vi "Begin.vi"() -> ()   [LabVIEW 2019]
doc: "Called before other user functions, this VI is expected to open initial I/O refnums, load in file data, and do all program initialization. Notice that the <B>error out</B> terminal is simply used for data flow. Wiring it to other structures or subVIs ensures that this VI runs first."
uses:
  <vilib>/Rock Robotics/WPI/Solenoid/WPI_SolenoidOpenSingle.vi
  <vilib>/Rock Robotics/WPI/RobotDrive/WPI_RobotDriveOpen4MotorWithSPARK.vi
  <vilib>/Rock Robotics/WPI/MotorControl/WPI_MotorControlOpen SPARK.vi
  <vilib>/Rock Robotics/WPI/MotorControl/WPI_MotorControlOpen TalonSRX.vi
  <vilib>/Rock Robotics/SystemInterfaces/DIO/FPGA_DIOPWMChannel.ctl
  <vilib>/Rock Robotics/WPI/Solenoid/WPI_SolenoidChannel.ctl
  <vilib>/Rock Robotics/WPI/Joystick/WPI_JoystickDeviceEnum.ctl
panel:
  in  "Shooting Motor 2 PWM Channel":T1
  in  "Shooting Motor 1 PWM Channel":T1
  in  "Peripherals Controller":T2
  in  "Drive Controller":T2
  in  "Transport Motor PWM Channel":T1
  in  "Intake Motor PWM Channel":T1
  in  "Pneumatics Control Module (0) 3":u8
  in  "Solenoid Channel 2":T3
  in  "Pneumatics Control Module (0) 2":u8
  in  "Solenoid Channel":T3
  in  "Pneumatics Control Module (0)":u8
  in  "Rear Camera Address":string="192.168.0.90"
  in  "Front Camera Address":string="192.168.0.90"
  in  "Front Right Motor Inverted":bool
  in  "Front Left Motor Inverted":bool
  in  "Rear Right Motor Inverted":bool
  in  "Rear Left Motor Inverted":bool
  in  "Front Right Motor":T1=enum."Invalid"
  in  "Front Left Motor":T1=enum."Invalid"
  in  "Rear Right Motor":T1=enum."Invalid"
  in  "Rear Left Motor":T1=enum."Invalid"
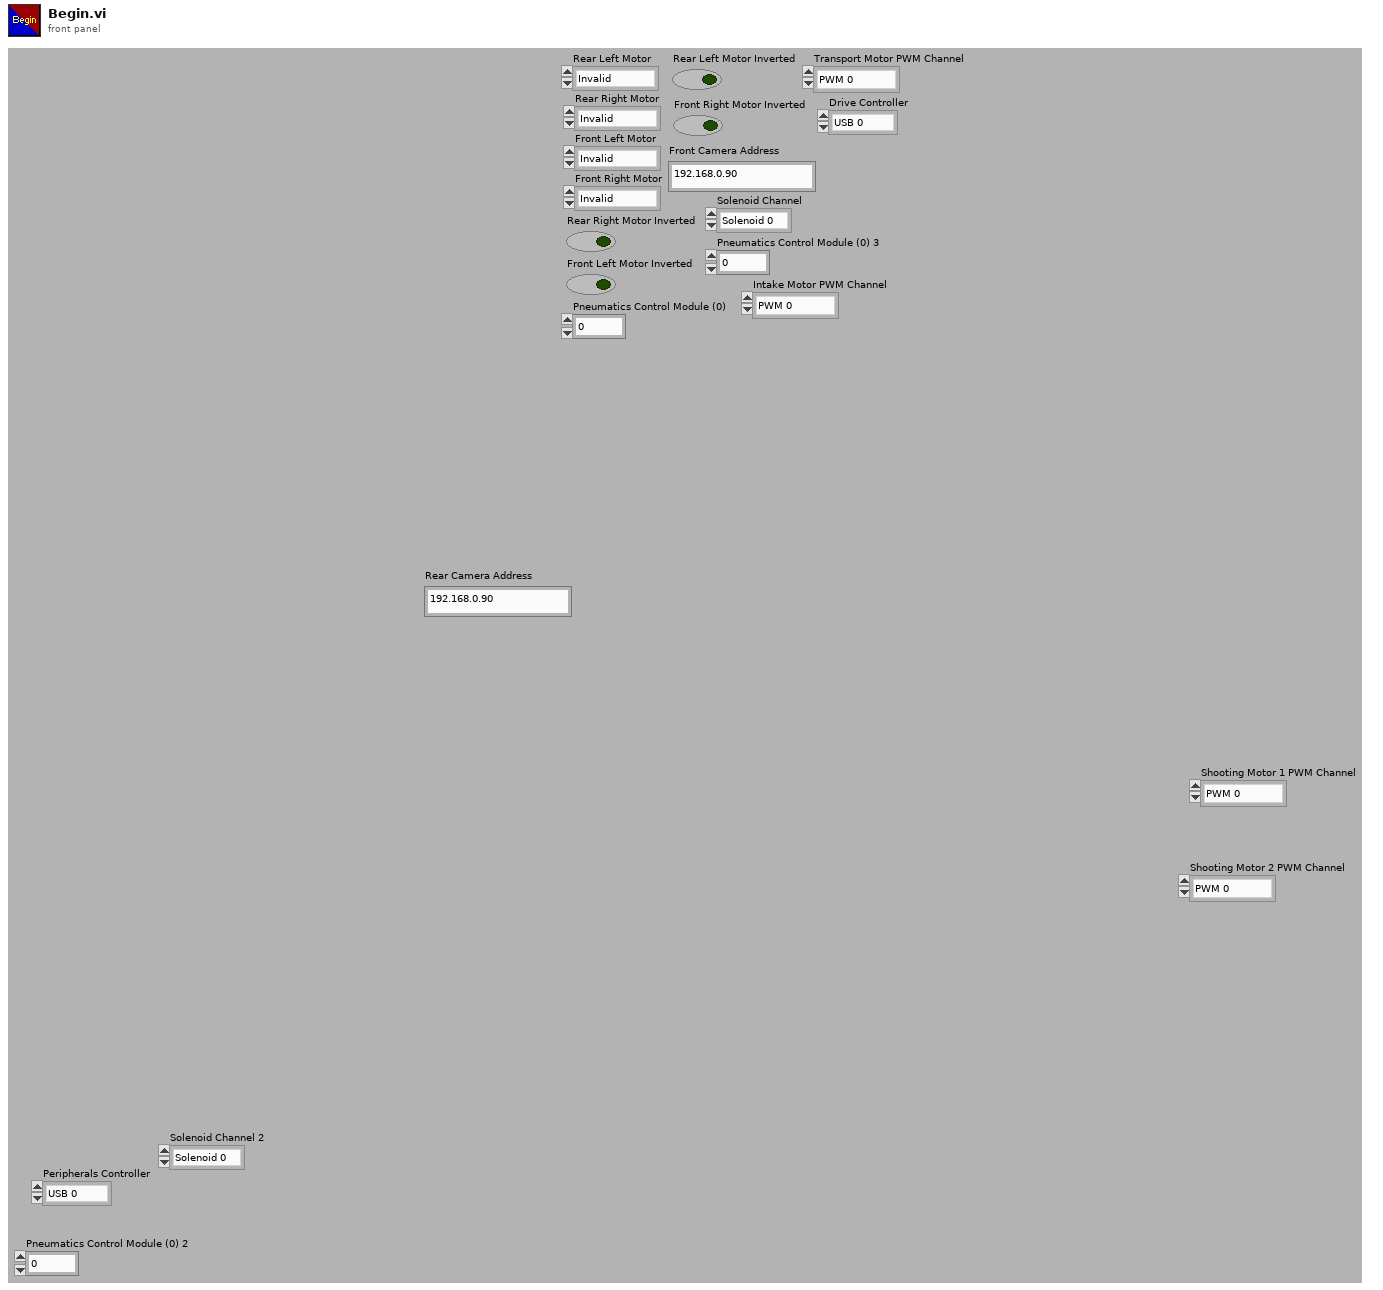
[diagram p1: front panel]
types:
  T1 = typedef "FPGA_DIOPWMChannel.ctl" = enum8{"PWM 0", "PWM 1", "PWM 2", "PWM 3", "PWM 4", "PWM 5", "PWM 6", "PWM 7", "PWM 8", "PWM 9", "PWM MXP 0", "PWM MXP 1", "PWM MXP 2", "PWM MXP 3", "PWM MXP 4", "PWM MXP 5", "PWM MXP 6", "PWM MXP 7", "PWM MXP 8", "PWM MXP 9", "Invalid"}
  T2 = typedef "WPI_JoystickDeviceEnum.ctl" = enum16{"USB 0", "USB 1", "USB 2", "USB 3", "USB 4", "USB 5"}
  T3 = typedef "WPI_SolenoidChannel.ctl" = enum8{"Solenoid 0", "Solenoid 1", "Solenoid 2", "Solenoid 3", "Solenoid 4", "Solenoid 5", "Solenoid 6", "Solenoid 7", "Invalid"}
  T4 = typedef "WPI_JoystickDevRef.ctl" = cluster{"Device":T2}
  T5 = typedef "WPI_RobotDriveDevRef.ctl" = cluster{"DevStatus":errorcluster, "Motors[]":T6[], "Square Inputs":bool, "Max Output":dbl}
  T6 = typedef "WPI_MotorControlDeviceRef.ctl" = cluster{"DeviceStatus":errorcluster, "Type":T7, "PWM":cluster{"PWM Channel":T1, "DeadBand":T8}, "CAN":cluster{"Device Number":u8, "SetOutput VI Ref":variant, "GetOutput VI Ref":variant, "Enable VI Ref":variant, "Disable VI Ref":variant, "Data":variant}, "Invert":bool, "DIO PWM":cluster{"PWM \"Enable\" Channel":T1, "DIOChannel":T9, "PWM Rate":dbl}}
  T7 = typedef "WPI_MotorControlType.ctl" = enum16{"PWM", "CAN", "DIO PWM"}
  T8 = typedef "WPI_PWMDeadband.ctl" = cluster{"Name":string, "maxPositivePwm":i32, "minPositivePwm":i32, "centerPwm":i32, "maxNegativePwm":i32, "minNegativePwm":i32, "angularRange":u16}
  T9 = typedef "FPGA_DIOChannel.ctl" = enum8{"DIO 0", "DIO 1", "DIO 2", "DIO 3", "DIO 4", "DIO 5", "DIO 6", "DIO 7", "DIO 8", "DIO 9", "DIO MXP 0", "DIO MXP 1", "DIO MXP 2", "DIO MXP 3", "DIO MXP 4", "DIO MXP 5", "DIO MXP 6", "DIO MXP 7", "DIO MXP 8", "DIO MXP 9", "DIO MXP 10", "DIO MXP 11", "DIO MXP 12", "DIO MXP 13", "DIO MXP 14", "DIO MXP 15", "SPI Port CS1", "SPI Port CS2", "SPI Port CS3", "SPI Port MISO", "SPI Port MOSI", "Invalid"}
  T10 = typedef "WPI_CameraDevRef.ctl" = cluster{"Camera Address":string, "CameraStatus":errorcluster}
  T11 = typedef "WPI_SolenoidDevRef.ctl" = cluster{"DevStatus":errorcluster, "Pneumatics Control Module":u8, "Forward Solenoid Channel":T3, "Reverse Solenoid Channel":T3}
  T12 = typedef "WPI_CompressorDevRef.ctl" = cluster{"DevStatus":errorcluster, "Pneumatics Control Module":u8}
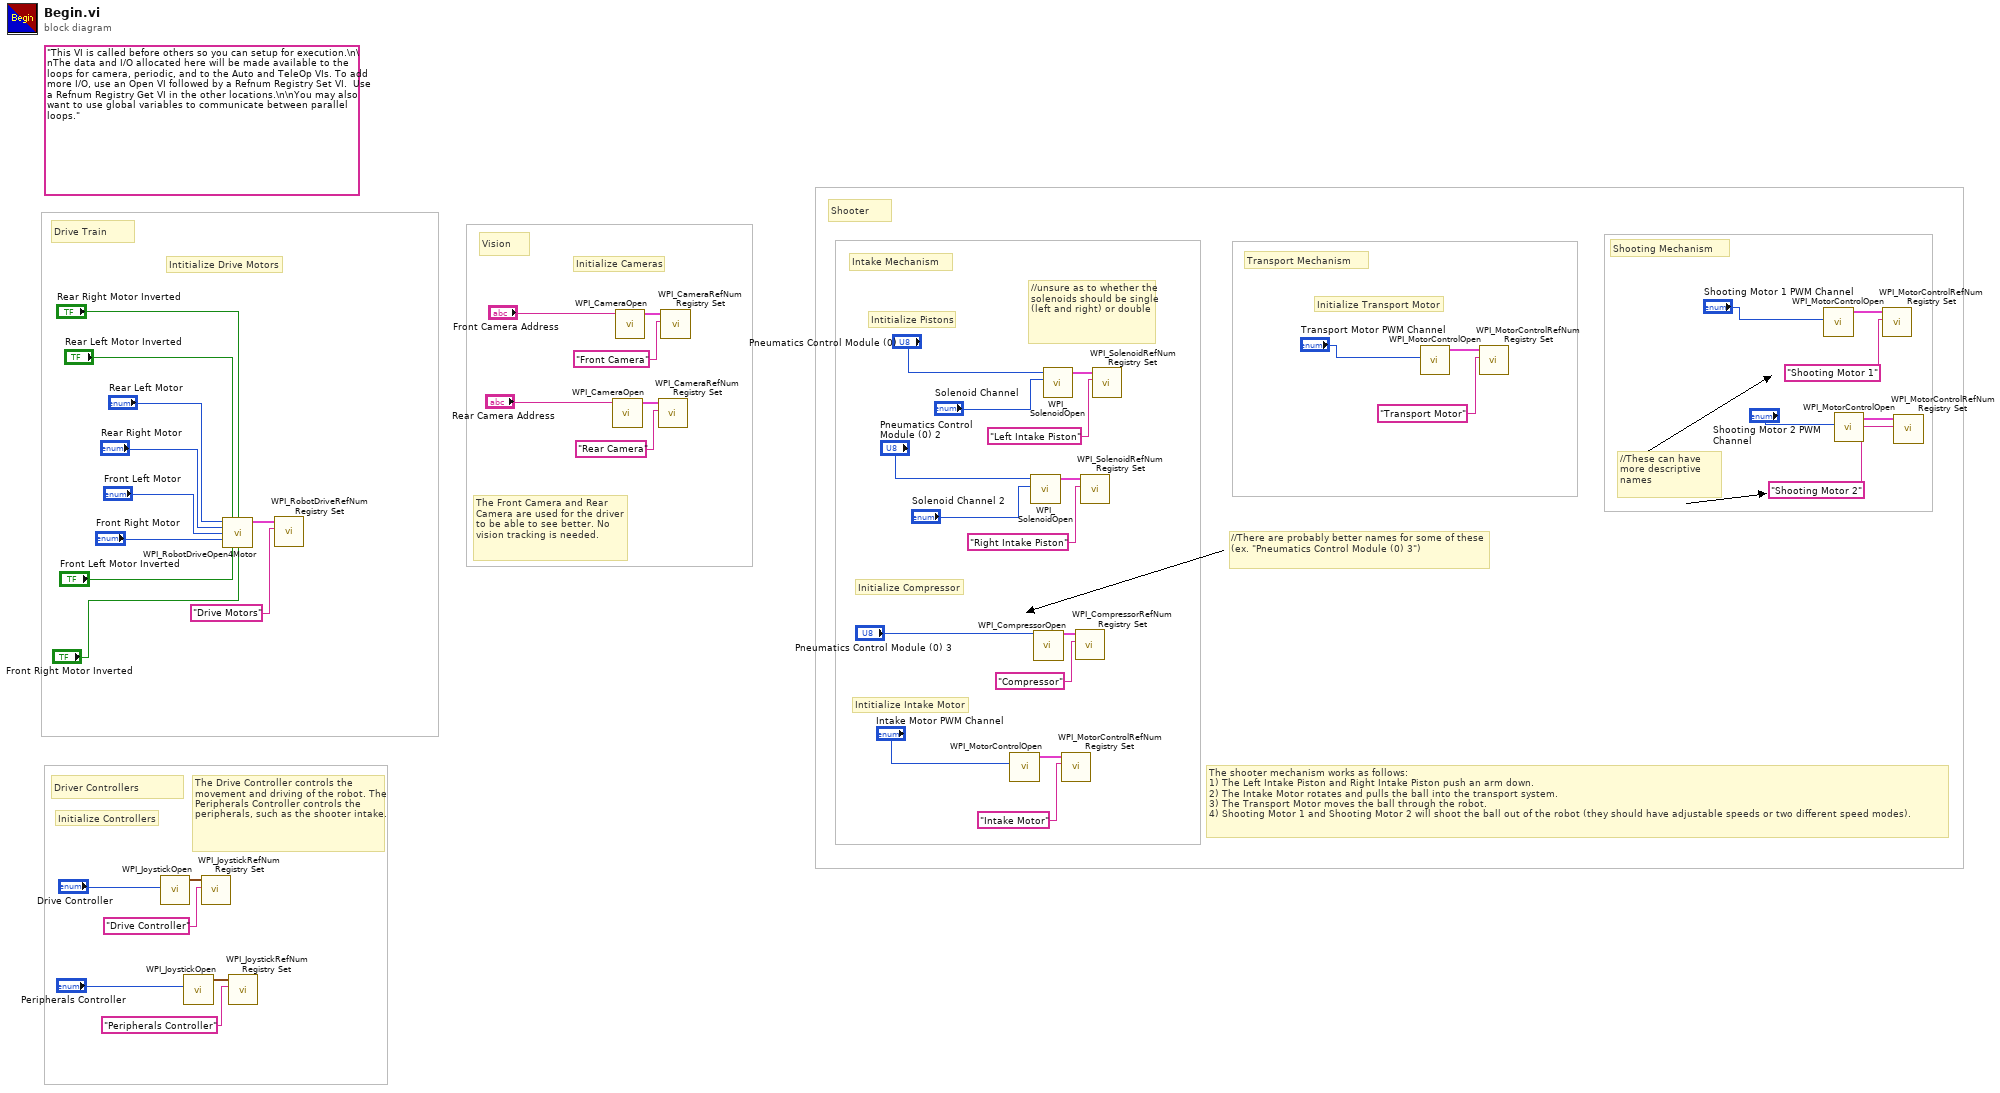
[diagram p0: block diagram]
diagram:
  (unwired) "This VI is called before others so you can setup for execution.\n\nThe data and I/O allocated here will be made available to the loops for camera, periodic, and to the Auto and TeleOp VIs. To add more I/O, use an Open VI followed by a Refnum Registry Set VI.  Use a Refnum Registry Get VI in the other locations.\n\nYou may also want to use global variables to communicate between parallel loops."
  # "Shooting Mechanism"
  # "//These can have more descriptive names"
  # "//unsure as to whether the solenoids should be single (left and right) or double"
  # "The shooter mechanism works as follows:\n1) The Left Intake Piston and Right Intake Piston push an arm down.\n2) The Intake Motor rotates and pulls the ball into the transport system.\n3) The Transport Motor moves the ball through the robot.\n4) Shooting Motor 1 and Shooting Motor 2 will shoot the ball out of the robot (they should have adjustable speeds or two different speed modes)."
  # "The Front Camera and Rear Camera are used for the driver to be able to see better. No vision tracking is needed."
  # "The Drive Controller controls the movement and driving of the robot. The Peripherals Controller controls the peripherals, such as the shooter intake."
  # "Initialize Controllers"
  # "Driver Controllers"
  # "//There are probably better names for some of these (ex. \"Pneumatics Control Module (0) 3\")"
  # "Transport Mechanism"
  # "Intake Mechanism"
  # "Shooter"
  # "Vision"
  # "Drive Train"
  # "Initialize Transport Motor"
  # "Intitialize Intake Motor"
  # "Initialize Compressor"
  # "Intitialize Pistons"
  # "Initialize Cameras"
  # "Intitialize Drive Motors"
  n1 = call <vilib>:"WPI_JoystickOpen.vi"("JoystickDevice"="Drive Controller") -> ("JoystickDevRef"=w12:T4)  [unwired: 10 in]
  n2 = call <vilib>:"WPI_JoystickOpen.vi"("JoystickDevice"="Peripherals Controller") -> ("JoystickDevRef"=w9:T4)  [unwired: 10 in]
  n3 = call <vilib>:"WPI_JoystickRefNum Registry Set.vi"("refnum name"="Drive Controller", "JoystickDevRef"=w12) -> ()  [unwired: 8 in, 2 out]
  n4 = call-poly <vilib>:"WPI_RobotDriveOpen4Motor.vi"("Rear Left Motor"="Rear Left Motor", "Rear Left Motor Inverted"="Rear Left Motor Inverted", "Rear Right Motor Inverted"="Rear Right Motor Inverted", "Rear Right Motor"="Rear Right Motor", "Front Left Motor"="Front Left Motor", "Front Right Motor"="Front Right Motor", "Front Left Motor Inverted"="Front Left Motor Inverted", "Front Right Motor Inverted"="Front Right Motor Inverted") -> ("RobotDriveDevRef"=w37:T5)  [unwired: 6 in, 1 out]
  n5 = call <vilib>:"WPI_JoystickRefNum Registry Set.vi"("refnum name"="Peripherals Controller", "JoystickDevRef"=w9) -> ()  [unwired: 8 in, 2 out]
  n6 = call <vilib>:"WPI_RobotDriveRefNum Registry Set.vi"("refnum name"="Drive Motors", "RobotDriveDevRef"=w37) -> ()  [unwired: 8 in, 2 out]
  n7 = call <vilib>:"WPI_CameraOpen.vi"("Camera Address"="Rear Camera Address") -> ("CameraDevRef"=w31:T10)  [unwired: 9 in, 1 out]
  n8 = call <vilib>:"WPI_CameraOpen.vi"("Camera Address"="Front Camera Address") -> ("CameraDevRef"=w34:T10)  [unwired: 9 in, 1 out]
  n9 = call <vilib>:"WPI_CameraRefNum Registry Set.vi"("refnum name"="Rear Camera", "CameraDevRef"=w31) -> ()  [unwired: 8 in, 2 out]
  n10 = call <vilib>:"WPI_CameraRefNum Registry Set.vi"("refnum name"="Front Camera", "CameraDevRef"=w34) -> ()  [unwired: 8 in, 2 out]
  n11 = call-poly <vilib>:"WPI_MotorControlOpen.vi"("PWM Channel"="Intake Motor PWM Channel") -> ("MotorControlDeviceRef"=w18:T6)  [unwired: 9 in, 1 out]
  n12 = call-poly <vilib>:"WPI_SolenoidOpen.vi"("Solenoid Channel"="Solenoid Channel 2", "Pneumatics Control Module (0)"="Pneumatics Control Module (0) 2") -> ("SolenoidDevRef"=w25:T11)  [unwired: 8 in, 1 out]
  n13 = call <vilib>:"WPI_CompressorOpen.vi"("Pneumatics Control Module (0)"="Pneumatics Control Module (0) 3") -> ("CompressorDevRef"=w21:T12)  [unwired: 13 in, 1 out]
  n14 = call-poly <vilib>:"WPI_SolenoidOpen.vi"("Solenoid Channel"="Solenoid Channel", "Pneumatics Control Module (0)"="Pneumatics Control Module (0)") -> ("SolenoidDevRef"=w29:T11)  [unwired: 8 in, 1 out]
  n15 = call <vilib>:"WPI_MotorControlRefNum Registry Set.vi"("refnum name"="Intake Motor", "MotorControlDevRef"=w18) -> ()  [unwired: 8 in, 2 out]
  n16 = call <vilib>:"WPI_CompressorRefNum Registry Set.vi"("refnum name"="Compressor", "CompressorDevRef"=w21) -> ()  [unwired: 8 in, 2 out]
  n17 = call <vilib>:"WPI_SolenoidRefNum Registry Set.vi"("refnum name"="Right Intake Piston", "SolenoidDevRef"=w25) -> ()  [unwired: 8 in, 2 out]
  n18 = call <vilib>:"WPI_SolenoidRefNum Registry Set.vi"("refnum name"="Left Intake Piston", "SolenoidDevRef"=w29) -> ()  [unwired: 8 in, 2 out]
  n19 = call-poly <vilib>:"WPI_MotorControlOpen.vi"("PWM Channel"="Transport Motor PWM Channel") -> ("MotorControlDeviceRef"=w14:T6)  [unwired: 9 in, 1 out]
  n20 = call <vilib>:"WPI_MotorControlRefNum Registry Set.vi"("refnum name"="Transport Motor", "MotorControlDevRef"=w14) -> ()  [unwired: 8 in, 2 out]
  n21 = call-poly <vilib>:"WPI_MotorControlOpen.vi"("PWM Channel"="Shooting Motor 1 PWM Channel") -> ("MotorControlDeviceRef"=w5:T6)  [unwired: 9 in, 1 out]
  n22 = call-poly <vilib>:"WPI_MotorControlOpen.vi"("PWM Channel"="Shooting Motor 2 PWM Channel") -> ("MotorControlDeviceRef"=w3:T6)  [unwired: 9 in, 1 out]
  n23 = call <vilib>:"WPI_MotorControlRefNum Registry Set.vi"("refnum name"="Shooting Motor 1", "MotorControlDevRef"=w5) -> ()  [unwired: 8 in, 2 out]
  n24 = call <vilib>:"WPI_MotorControlRefNum Registry Set.vi"("refnum name"="Shooting Motor 2", "MotorControlDevRef"=w3) -> ()  [unwired: 8 in, 2 out]
